vi "Math_Add_FXP.vi"(1 "y":fxp<+/-,32,16> format="%#_32g", 2 "x":fxp<+/-,32,16> format="%#_32g") -> (0 "x*y":fxp<+/-,32,16>)   [LabVIEW 2020]
uses:
  <vilib>/rvi/FXPMathLib/FxpAdd/XNode/nifxpmath_Add.xnode
  <vilib>/rvi/FXPMathLib/sim/FxpSim.dll
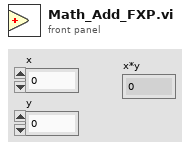
[diagram p1: front panel]
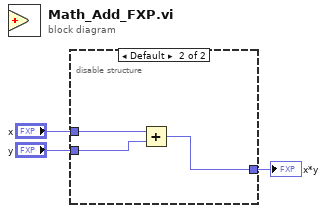
[diagram p0: block diagram]
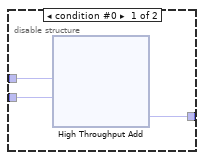
[diagram p2: hidden frame]
diagram:
  n1 = disable-structure shown="Default" {
    disable-tunnel: "y" -> [w6 w8]
    disable-tunnel: [w5 w7] -> w2
    disable-tunnel: "x" -> [w4 w9]
    frame condition #0 {
      n2 = xnode "High Throughput Add"("x"=w4, "y"=w6) -> ("x+y"=w5:fxp<+/-,32,16>)
    }
    frame condition #1 (active) {
      n3 = Add(x=w9, y=w8) -> (x+y=w7:fxp<+/-,32,16>)
    }
  }
  "x*y" <- w2
